vi "GetCellStrColor.vi"(7 "Color":u32, 8 "error in (no error)":errorcluster, 10 "Hdr Name":T1, 11 "Strain in":refnum<class "Strain.lvclass">) -> (0 "error out":errorcluster, 1 "Cell String":string, 2 "Cell Color":u32, 3 "Strain out":refnum<class "Strain.lvclass">)   [LabVIEW 2018, in "Measurement Channels.lvlib" / "Strain.lvclass"]
uses:
  Strain.lvclass
  Common/Controls/HeaderNames.ctl
  SubVIs Table/Custom Ctls Table/ge_ColType.ctl
  Strain.lvclass/Strain.ctl
  Class Channel/Channel.lvclass
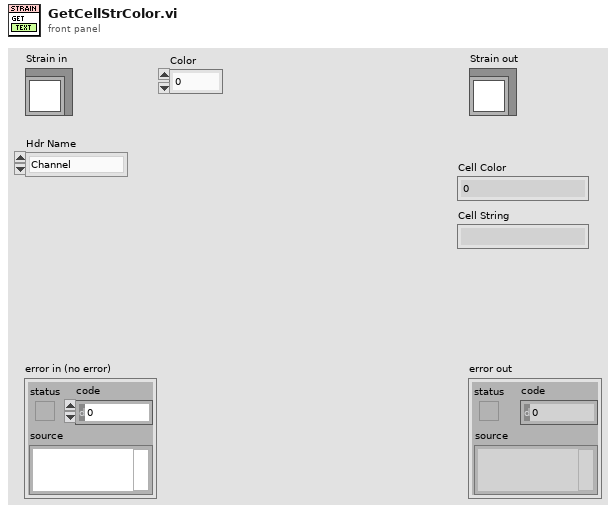
[diagram p1: front panel]
types:
  T1 = typedef "HeaderNames.ctl" = enum16{"Channel", "Device", "Spacer", "Description", "MB", "Range", "Terminal", "Coupling", "Thresh (V)", "Pulse/Rev", "Slope", "Min EU", "Min RPM", "mV/EU", "Iex", "Temp Units", "Type", "CJC Src", "CJC Val", "Ro", "Wire Cfg", "Strain Mode", "Vex", "Bridge Type", "GF", "Gauge Res", "Poisson", "Lead Res", "Init Strain", "GAF", "Scale", "Offset", "Unit (EU)", "dB?", "dB Ref", "Cal Mag", "Cal Units", "Max Temp", "Min Temp", "Max Strain", "Min Strain"}
  T2 = typedef "ge_ColType.ctl" = enum16{"Volts", "Amps", "Ohms", "TermCfg", "WireCfg", "Coup", "Slope", "Iex", "CalUnits", "ThrmUnits", "ThrmType", "CJCSrc", "BrdgType", "Strn Mode", "RTDType"}
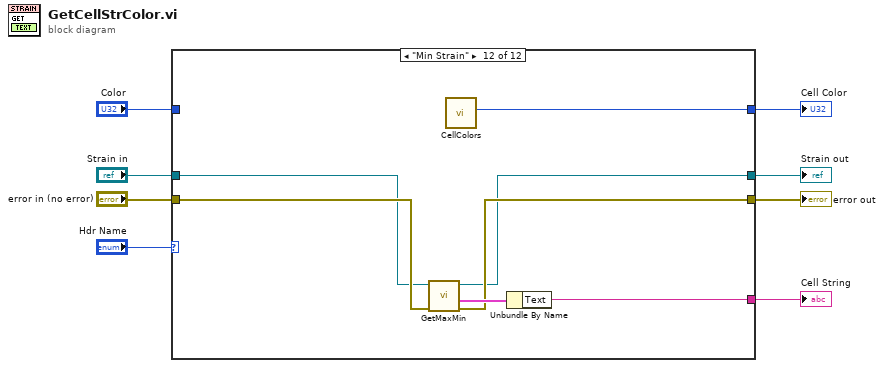
[diagram p0: block diagram]
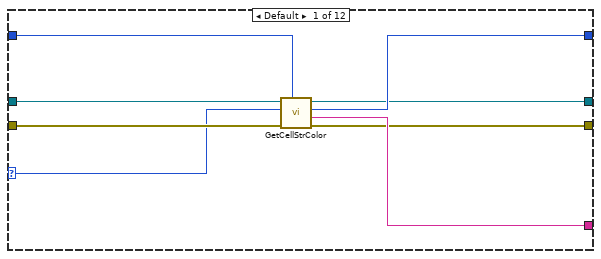
[diagram p2: hidden frame]
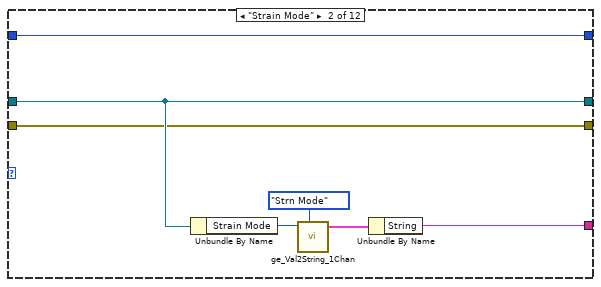
[diagram p3: hidden frame]
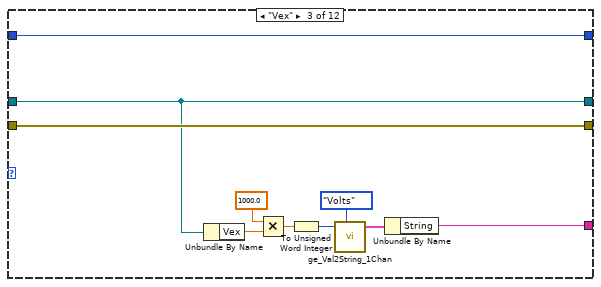
[diagram p4: hidden frame]
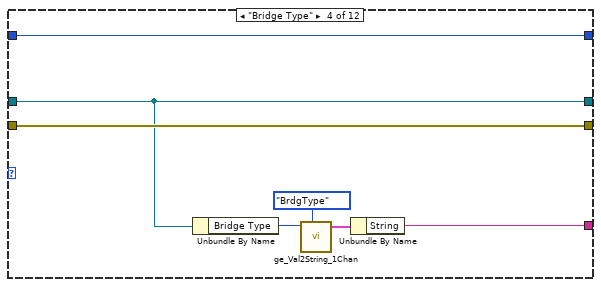
[diagram p5: hidden frame]
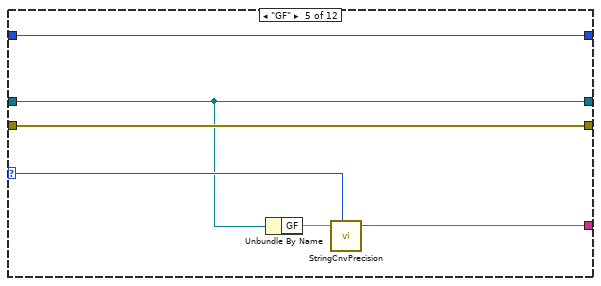
[diagram p6: hidden frame]
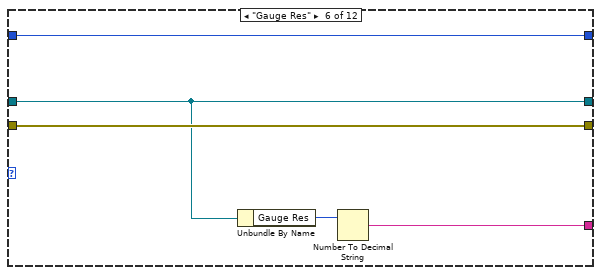
[diagram p7: hidden frame]
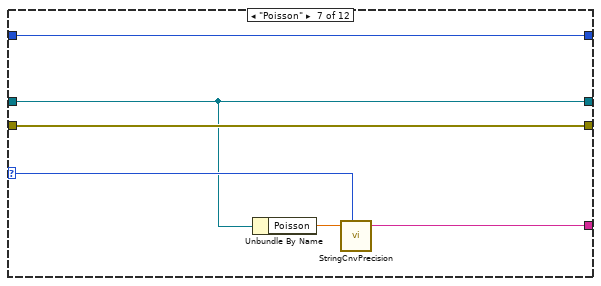
[diagram p8: hidden frame]
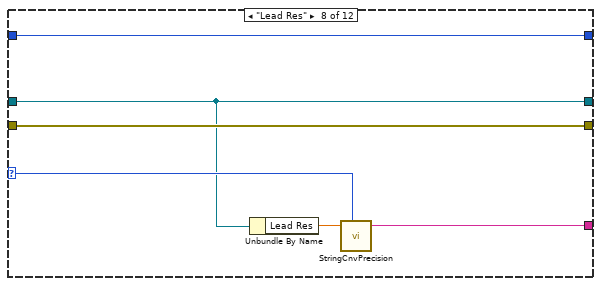
[diagram p9: hidden frame]
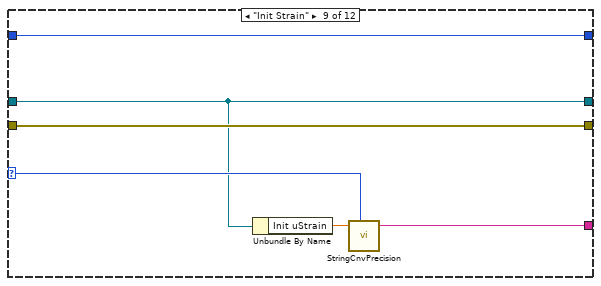
[diagram p10: hidden frame]
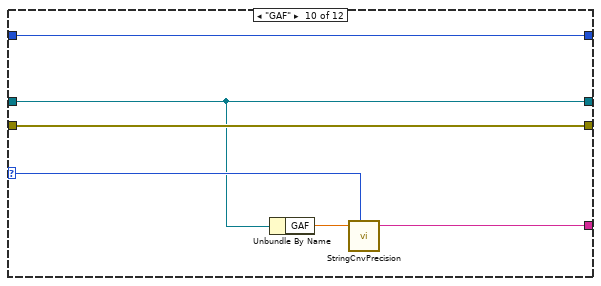
[diagram p11: hidden frame]
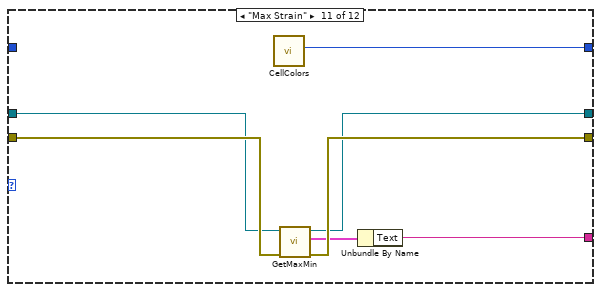
[diagram p12: hidden frame]
diagram:
  n1 = case shown="\"Min Strain\"" "Hdr Name" {
    selector: "Hdr Name" -> [w9 _ _ _ w44 _ w56 w62 w68 w74 _ _]
    tunnel: [w15 w21 w31 w38 w45 w51 w55 w61 w67 w73 w76 w83] -> w1
    tunnel: [w16 w19 w26 w36 w43 w49 w54 w60 w66 w72 w82 w89] -> w2
    tunnel: "Color" -> [w10 w19 w26 w36 w43 w49 w54 w60 w66 w72 _ _]
    tunnel: "Strain in" -> [w14 w18 w24 w34 w41 w47 w52 w58 w64 w70 w79 w84]
    tunnel: [w13 w18 w24 w34 w41 w47 w52 w58 w64 w70 w78 w85] -> w7
    tunnel: "error in (no error)" -> [w12 w17 w25 w35 w42 w48 w53 w59 w65 w71 w81 w87]
    tunnel: [w11 w17 w25 w35 w42 w48 w53 w59 w65 w71 w80 w86] -> w5
    frame Default {
      n2 = call-parent "GetCellStrColor.vi"("Color"=w10, "error in (no error)"=w12, "Hdr Name"=w9, "Channel in"=w14) -> ("error out"=w11:errorcluster, "Cell String"=w15:string, "Cell Color"=w16:u32, "Channel out"=w13:refnum<class "Strain.lvclass">)  [unwired: 4 in]
    }
    frame "Strain Mode" {
      n3 = Unbundle By Name(w18) -> ("Strain Mode"=w20:u16)
      n4 = call "ge_Val2String_1Chan.vi"("Value"=w20, "ColType"=ge_ColType."Strn Mode") -> ("String and Val"=w22:cluster{"String":string, "Value":u16})  [unwired: 5 in]
      n5 = Unbundle By Name(w22) -> ("String"=w21:string)
    }
    frame "Vex" {
      n6 = Unbundle By Name(w24) -> ("Vex"=w29:dbl)
      n7 = Multiply(x=1000.0, y=w29) -> (x*y=w30:dbl)
      n8 = To Unsigned Word Integer(number=w30) -> (unsigned 16bit integer=w27:u16)
      n9 = call "ge_Val2String_1Chan.vi"("Value"=w27, "ColType"=ge_ColType."Volts") -> ("String and Val"=w32:cluster{"String":string, "Value":u16})  [unwired: 5 in]
      n10 = Unbundle By Name(w32) -> ("String"=w31:string)
    }
    frame "Bridge Type" {
      n11 = Unbundle By Name(w34) -> ("Bridge Type"=w37:u16)
      n12 = call "ge_Val2String_1Chan.vi"("Value"=w37, "ColType"=ge_ColType."BrdgType") -> ("String and Val"=w39:cluster{"String":string, "Value":u16})  [unwired: 5 in]
      n13 = Unbundle By Name(w39) -> ("String"=w38:string)
    }
    frame "GF" {
      n14 = Unbundle By Name(w41) -> ("GF"=w46:dbl)
      n15 = call "StringCnvPrecision.vi"("Number"=w46, "Header"=w44) -> ("Float String"=w45:string)  [unwired: 5 in]
    }
    frame "Gauge Res" {
      n16 = Unbundle By Name(w47) -> ("Gauge Res"=w50:i32)
      n17 = Number To Decimal String(number=w50) -> (decimal integer string=w51:string)  [unwired: 1 in]
    }
    frame "Poisson" {
      n18 = Unbundle By Name(w52) -> ("Poisson"=w57:dbl)
      n19 = call "StringCnvPrecision.vi"("Number"=w57, "Header"=w56) -> ("Float String"=w55:string)  [unwired: 5 in]
    }
    frame "Lead Res" {
      n20 = Unbundle By Name(w58) -> ("Lead Res"=w63:dbl)
      n21 = call "StringCnvPrecision.vi"("Number"=w63, "Header"=w62) -> ("Float String"=w61:string)  [unwired: 5 in]
    }
    frame "Init Strain" {
      n22 = Unbundle By Name(w64) -> ("Init uStrain"=w69:dbl)
      n23 = call "StringCnvPrecision.vi"("Number"=w69, "Header"=w68) -> ("Float String"=w67:string)  [unwired: 5 in]
    }
    frame "GAF" {
      n24 = Unbundle By Name(w70) -> ("GAF"=w75:dbl)
      n25 = call "StringCnvPrecision.vi"("Number"=w75, "Header"=w74) -> ("Float String"=w73:string)  [unwired: 5 in]
    }
    frame "Max Strain" {
      n26 = call "CellColors.vi"() -> ("Disabled"=w82:u32)  [unwired: 8 in, 3 out]
      n27 = call-dynamic "GetMaxMin.vi"("error in (no error)"=w81, "Strain in"=w79) -> ("error out"=w80:errorcluster, "Max"=w77:cluster{"Value":dbl, "Text":string}, "Strain out"=w78:refnum<class "Strain.lvclass">)  [unwired: 6 in, 1 out]
      n28 = Unbundle By Name(w77) -> ("Text"=w76:string)
    }
    frame "Min Strain" {
      n29 = call-dynamic "GetMaxMin.vi"("error in (no error)"=w87, "Strain in"=w84) -> ("error out"=w86:errorcluster, "Min"=w88:cluster{"Value":dbl, "Text":string}, "Strain out"=w85:refnum<class "Strain.lvclass">)  [unwired: 6 in, 1 out]
      n30 = call "CellColors.vi"() -> ("Disabled"=w89:u32)  [unwired: 8 in, 3 out]
      n31 = Unbundle By Name(w88) -> ("Text"=w83:string)
    }
  }
  "error out" <- w5
  "Strain out" <- w7
  "Cell String" <- w1
  "Cell Color" <- w2
